vi "用户下子.vi"(0 "当前棋盘状态":i32[][](array[numeric]), 1 "控制数组":bool[][](array[boolean])) -> (4 "当前棋盘状态":i32[][](array[numeric]), 6 "当前点可下?":bool, 8 "行":sgl, 10 "列":i16)   [LabVIEW 2018]
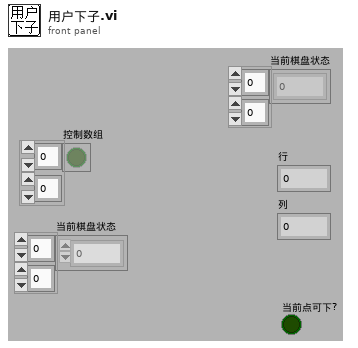
[diagram p1: front panel]
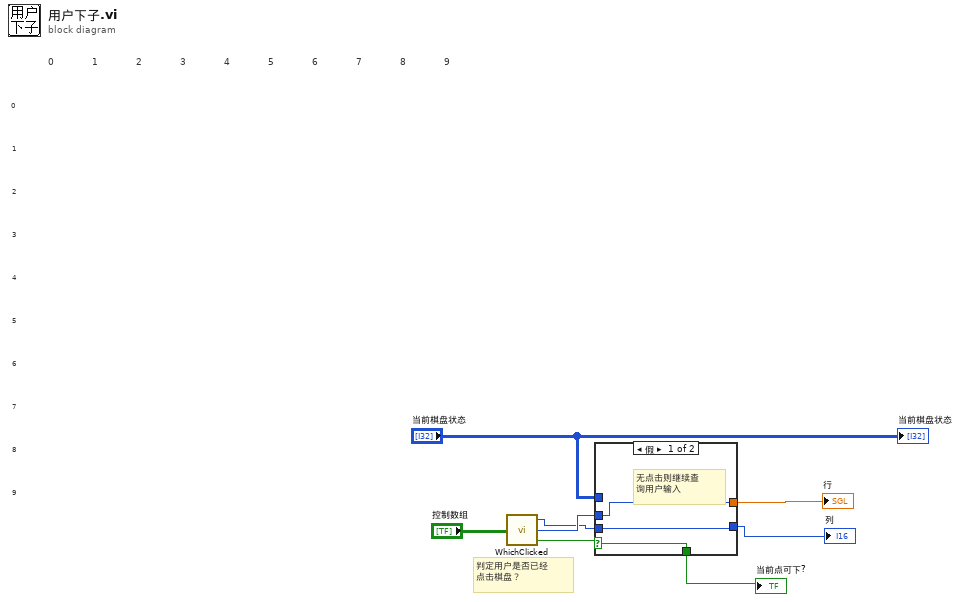
[diagram p0: block diagram]
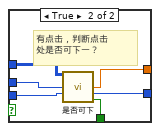
[diagram p2: hidden frame]
diagram:
  # "判定用户是否已经\n点击棋盘？"
  # "9"
  # "8"
  # "7"
  # "6"
  # "5"
  # "4"
  # "3"
  # "2"
  # "1"
  # "0"
  # "9"
  # "8"
  # "7"
  # "6"
  # "5"
  # "4"
  # "3"
  # "2"
  # "1"
  # "0"
  n1 = call "WhichClicked.vi"("Buttons"="控制数组") -> ("X"=w1:i32, "Y"=w2:i32, "OneClicked?"=w6:bool)
  n2 = case shown="假" w6 {
    selector: w6 -> [w9 _]
    tunnel: "当前棋盘状态" -> [_ w17]
    tunnel: w2 -> [w11 w16]
    tunnel: w1 -> [w10 w15]
    tunnel: [w11 w14] -> w8
    tunnel: [w9 w13] -> w5
    tunnel: [w10 w12] -> w4
    frame False {
      # "无点击则继续查\n询用户输入"
    }
    frame True {
      # "有点击，判断点击\n处是否可下一？"
      n3 = call "是否可下.vi"("当前棋盘状态"=w17, "行"=w16, "列"=w15) -> ("行"=w14:sgl, "列"=w12:i16, "当前点可下?"=w13:bool)  [unwired: 9 in, 1 out]
    }
  }
  "行" <- w8
  "列" <- w4
  "当前点可下?" <- w5
  "当前棋盘状态" <- "当前棋盘状态"
